vi "Write to device.vi"(5 "DataArray":u16[](array[numeric]), 7 "StartAddr":u16, 8 "error in (no error)":errorcluster, 10 "Address":T1, 11 "MB class in":refnum<class "MB class.lvclass">) -> (0 "error out":errorcluster, 2 "Address Out":T1, 3 "MB class out":refnum<class "MB class.lvclass">)   [LabVIEW 2020, in "MB class.lvclass"]
uses:
  MB class.lvclass
  MB class.lvclass/MB class.ctl
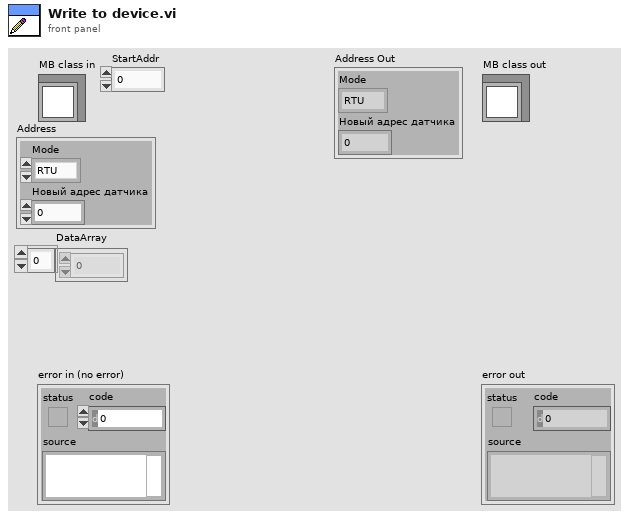
[diagram p1: front panel]
types:
  T1 = cluster{"Mode":enum16{"RTU", "ASCII"}, "Новый адрес датчика":u16}
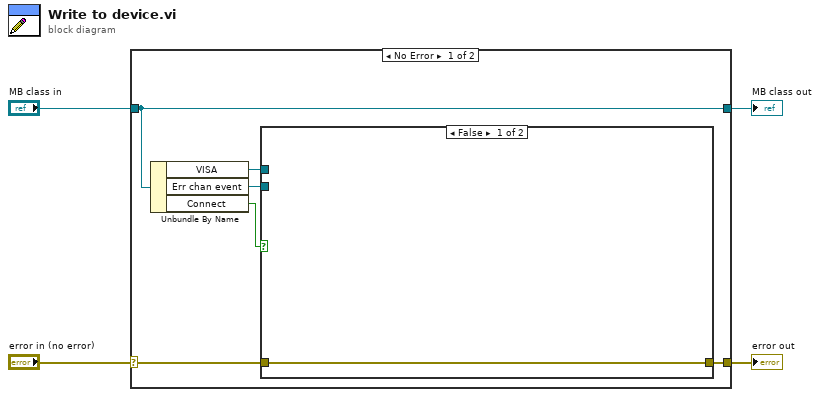
[diagram p0: block diagram]
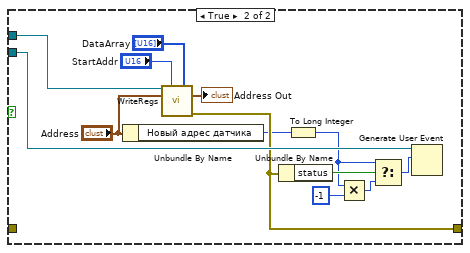
[diagram p2: hidden frame]
diagram:
  n1 = case shown="No Error" "error in (no error)" {
    selector: "error in (no error)" -> [w5 w26]
    tunnel: [w7 w26] -> w3
    tunnel: [w10 w25] -> w1
    tunnel: "MB class in" -> [w10 w25]
    frame No Error {
      n2 = Unbundle By Name(w10) -> ("VISA"=w9:refnum<visa-resource-name>, "Err chan event"=w8:refnum<user-event>, "Connect"=w6:bool)
      n3 = case shown="False" w6 {
        tunnel: w9 -> [_ w24]
        tunnel: w8 -> [_ w20]
        tunnel: [w11 w18] -> w7
        tunnel: w5 -> [w11 _]
        frame False {
        }
        frame True {
          n4 = Unbundle By Name("Address") -> ("Новый адрес датчика"=w15:u16)
          n5 = call "WriteRegs.vi"("VISA Refnum in"=w24, "StartAddr"="StartAddr", "DataArray"="DataArray", "Cluster"="Address") -> ("Cluster Out"=→"Address Out":T1, "error out"=w18:errorcluster)  [unwired: 9 in, 1 out]
          n6 = Unbundle By Name(w18) -> ("status"=w17:bool)
          n7 = To Long Integer(number=w15) -> (32bit integer=w14:i32)
          n8 = Multiply(x=w14, y=-1) -> (x*y=w12:i32)
          n9 = Select(t=w14, s=w17, f=w12) -> (s? t:f=w16:i32)
          n10 = Generate User Event(user event=w20, event data cluster=w16) -> ()  [unwired: 2 in, 2 out]
        }
      }
    }
    frame Error {
    }
  }
  "error out" <- w3
  "MB class out" <- w1
